vi "Set_Mode.vi"(6 "Error In":errorcluster, 7 "Mode":T1(ring), 8 "Node":u8, 9 "Serial In":refnum<visa-resource-name>) -> (0 "Error Out":errorcluster, 3 "Serial Out":refnum<visa-resource-name>)   [LabVIEW 2019]
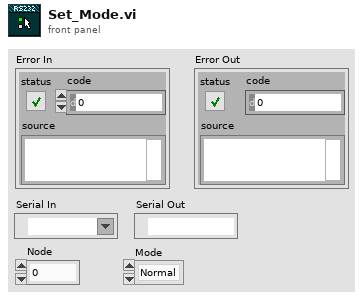
[diagram p1: front panel]
types:
  T1 = enum16{"Normal", "Stepper Motor", "Gearing", "Voltage Regulator", "Current Control (Preset Direction)", "Current Control (Sign Direction)", "IxR Control"}
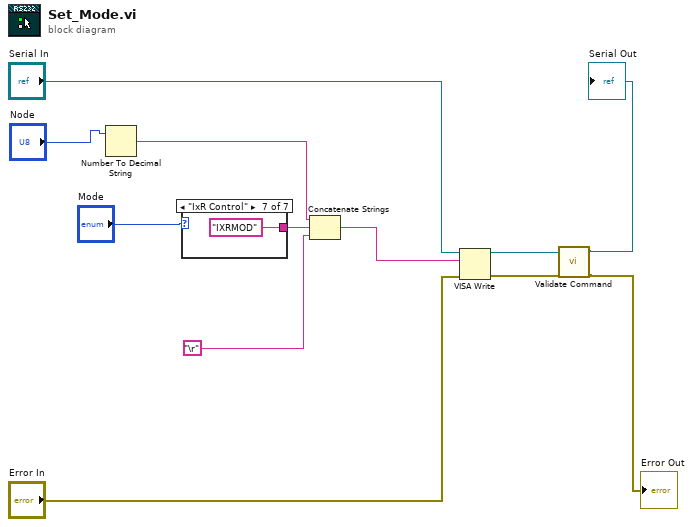
[diagram p0: block diagram]
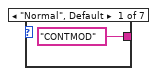
[diagram p2: hidden frame]
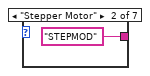
[diagram p3: hidden frame]
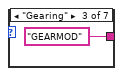
[diagram p4: hidden frame]
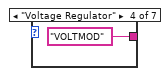
[diagram p5: hidden frame]
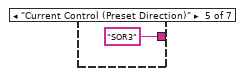
[diagram p6: hidden frame]
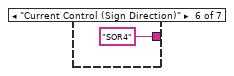
[diagram p7: hidden frame]
diagram:
  n1 = Number To Decimal String(number="Node") -> (decimal integer string=w9:string)  [unwired: 1 in]
  n2 = case shown="\"IxR Control\"" "Mode" {
    tunnel: ["CONTMOD" ("string") "STEPMOD" ("string") "GEARMOD" ("string") "VOLTMOD" ("string") "SOR3" ("string") "SOR4" ("string") "IXRMOD" ("string")] -> w7
    frame "Normal", Default {
    }
    frame "Stepper Motor" {
    }
    frame "Gearing" {
    }
    frame "Voltage Regulator" {
    }
    frame "Current Control (Preset Direction)" {
    }
    frame "Current Control (Sign Direction)" {
    }
    frame "IxR Control" {
    }
  }
  n3 = Concatenate Strings(w9, w7, "\r") -> (w8:string)
  n4 = VISA Write(VISA resource name="Serial In", write buffer=w8, error in (no error)="Error In") -> (VISA resource name out=w5:refnum<visa-resource-name>, error out=w4:errorcluster)  [unwired: 1 out]
  n5 = call "Validate Command.vi"("error in (no error)"=w4, "Serial in"=w5) -> ("error out"=→"Error Out":errorcluster, "Serial Out"=→"Serial Out":refnum<visa-resource-name>)  [unwired: 3 in, 1 out]
